vi "xPCScSoftTrigger.vi"(2 "error in (no error)":errorcluster, 3 "scope":i32, 4 "port":i32) -> (0 "error out":errorcluster, 1 "port copy":i32)   [LabVIEW 2018]
uses:
  XPCAPI.DLL
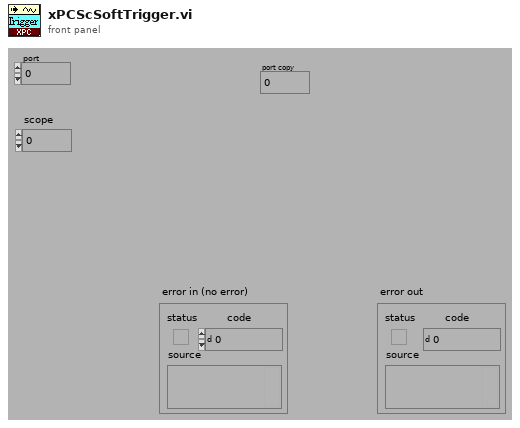
[diagram p1: front panel]
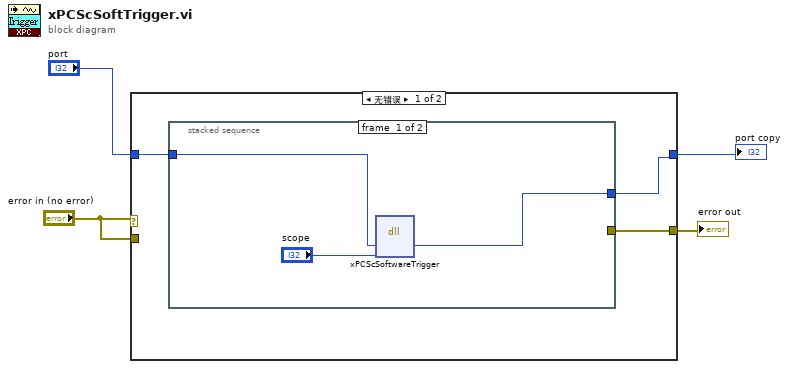
[diagram p0: block diagram]
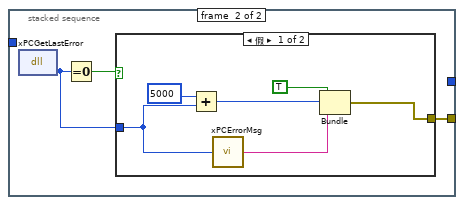
[diagram p2: hidden frame]
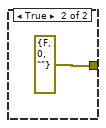
[diagram p3: hidden frame]
diagram:
  n1 = case shown="无错误" "error in (no error)" {
    tunnel: [w7 w22] -> w4
    tunnel: "error in (no error)" -> [_ w22]
    tunnel: "port" -> [w6 w21]
    tunnel: [w5 w21] -> w1
    frame No Error {
      n2 = stacked-sequence {
        tunnel: [w8 _] -> w5
        tunnel: [_ w11] -> w7
        tunnel: w6 -> [w9 _]
        frame #0 {
          n3 = dll-call lib="PTH2Iabs CUsers\nyuchengxinDesktop上下位机联机测试\nxpcapi.dll" fn="xPCScSoftwareTrigger" label="Call Library Function"("port"=w9, "scope"="scope") -> ("port"=w8:i32)  [unwired: 5 in, 2 out]
        }
        frame #1 {
          n4 = dll-call lib="PTH2Iabs CUsers\nyuchengxinDesktop上下位机联机测试\nxpcapi.dll" fn="xPCGetLastError"() -> (w12:i32)  [unwired: 3 in, 2 out]
          n5 = Equal To 0?(x=w12) -> (x = 0?=w13:bool)
          n6 = case shown="假" w13 {
            tunnel: w12 -> [w15 _]
            tunnel: [w16 errorcluster {"status"=FALSE, "code"=0, "source"=""} ("error out")] -> w11
            frame False {
              n7 = Add(x=5000 ("y"), y=w15) -> (x+y=w18:i32)
              n8 = call "xPCErrorMsg.vi"("error number"=w15) -> ("ErrorMsg"=w17:string)
              n9 = Bundle(TRUE, w18, "ErrorMsg"=w17) -> (w16:cluster{bool, i32, "ErrorMsg":string})  [unwired: 1 in]
            }
            frame True {
            }
          }
        }
      }
    }
    frame Error {
    }
  }
  "port copy" <- w1
  "error out" <- w4
